vi "Median Filter.vi"(9 "right rank":i32=-1, 10 "left rank":i32=2, 11 "X":dbl[](array[numeric])) -> (0 "error":i32, 3 "Filtered X":dbl[](array[numeric]))   [LabVIEW 2014, in "NI_AALBase.lvlib"]
doc: "Applies a median filter of rank to the input sequence <B>X</B>, where rank is <B>right rank</B> if <B>right rank</B> is greater than zero, or <B>left rank</B> if <B>right rank</B> is less than zero."
uses:
  NI_AALBase.lvlib
  lvanlys.dll
panel:
  # "Median Filter"
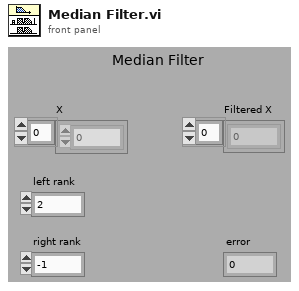
[diagram p1: front panel]
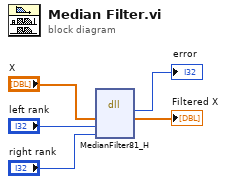
[diagram p0: block diagram]
diagram:
  n1 = dll-call lib="C:/Program Files (x86)/National Instruments/LabVIEW 2014/resource/lvanlys.*" fn="MedianFilter81_H"("xHandle"="X", "left rank"="left rank", "right rank"="right rank") -> (→"error":i32, "xHandle"=→"Filtered X":dbl[])  [unwired: 5 in, 2 out]
